vi "Initialise.vi"(8 "error in (no error)":errorcluster, 9 "Current Loop Rate (usec)":u32, 10 "frame":string="/world", 11 "MF3 in":refnum<class "MF3.lvclass">) -> (0 "error out":errorcluster, 3 "MF3 out":refnum<class "MF3.lvclass">)   [LabVIEW 2011, in "MF3.lvclass"]
uses:
  MF3.lvclass
  Controls/Drive Status.ctl
  <vilib>/LabVIEW Targets/FPGA/cRIO/cRIO-9505/controls.llb/_nicrio_cRIO-9505_DriveStatus.ctl
  MF3.lvclass/MF3.ctl
  <vilib>/FPGAPlugInAG/NI 9157/niLvFpga_Open_NI 9157.vi
  <vilib>/Utility/error.llb/Error Cluster From Error Code.vi
  <vilib>/rvi/errors/niLvFpgaAdjustHostInterfaceError.vi
  <vilib>/rvi/interface/nirviOpenFPGA/nirviOpenFPGA.xnode
  FPGA Bitfiles/MotorsInterface.lvbitx
  <vilib>/rvi/interface/nirviReadWriteControl/nirviReadWriteControl.xnode
  Finger/Finger.lvclass
  NiFpgaLv.dll
panel:
  out "Motors Status":T1[](array[typedef])=[{"Status"=enum."Enabled", "Vsup Present"=FALSE, "Drive Fault"=FALSE, "Temp Fault"=FALSE}, {"Status"=enum."Enabled", "Vsup Present"=FALSE, "Drive Fault"=FALSE, "Temp Fault"=FALSE}, {"Status"=enum."Enabled", "Vsup Present"=FALSE, "Drive Fault"=FALSE, "Temp Fault"=FALSE}, {"Status"=enum."Enabled", "Vsup Present"=FALSE, "Drive Fault"=FALSE, "Temp Fault"=FALSE}, {"Status"=enum."Enabled", "Vsup Present"=FALSE, "Drive Fault"=FALSE, "Temp Fault"=FALSE}, {"Status"=enum."Enabled", "Vsup Present"=FALSE, "Drive Fault"=FALSE, "Temp Fault"=FALSE}, {"Status"=enum."Enabled", "Vsup Present"=FALSE, "Drive Fault"=FALSE, "Temp Fault"=FALSE}, {"Status"=enum."Enabled", "Vsup Present"=FALSE, "Drive Fault"=FALSE, "Temp Fault"=FALSE}, {"Status"=enum."Enabled", "Vsup Present"=FALSE, "Drive Fault"=FALSE, "Temp Fault"=FALSE}, {"Status"=enum."Enabled", "Vsup Present"=FALSE, "Drive Fault"=FALSE, "Temp Fault"=FALSE}]
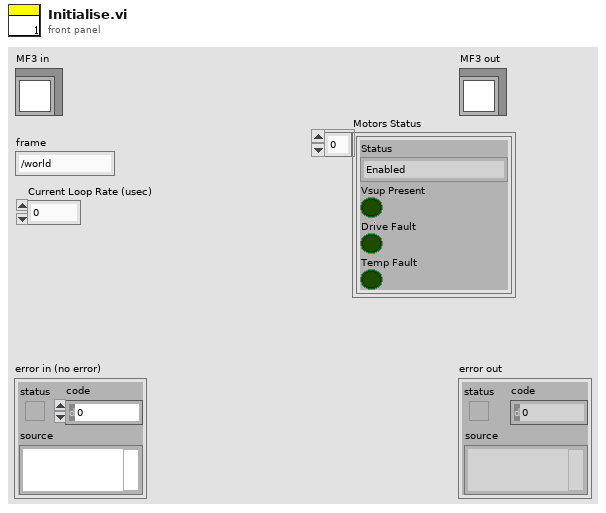
[diagram p1: front panel]
types:
  T1 = typedef "Drive Status.ctl" = cluster{"Status":T2, "Vsup Present":bool, "Drive Fault":bool, "Temp Fault":bool}
  T2 = typedef "_nicrio_cRIO-9505_DriveStatus.ctl" = enum8{"Enabled", "Disabled", "Disabled by Drive Fault", "Disabled by Temp. Fault", "Disabled by E-Stop", "Unknown"}
  T3 = typedef "Dynamic Parameters.ctl" = cluster{"gear_ratios":sgl[]}
  T4 = typedef "NI_Robotics_Link.lvclass/Joint Type.ctl" = enum16{"Revolute", "Prismatic"}
  T5 = typedef "5-bar Side.ctl" = enum16{"Left", "Right"}
  T6 = cluster{"Thumb":cluster{"k":sgl[][], "p":sgl[][], "T0":sgl[][], "types":T4[], "side":T5}, "Middle":cluster{"k":sgl[][], "p":sgl[][], "T0":sgl[][], "types":T4[], "side":T5}, "Index":cluster{"k":sgl[][], "p":sgl[][], "T0":sgl[][], "types":T4[], "side":T5}}
  T7 = cluster{"k":sgl[][], "p":sgl[][], "T0":sgl[][], "types":T4[], "side":T5}
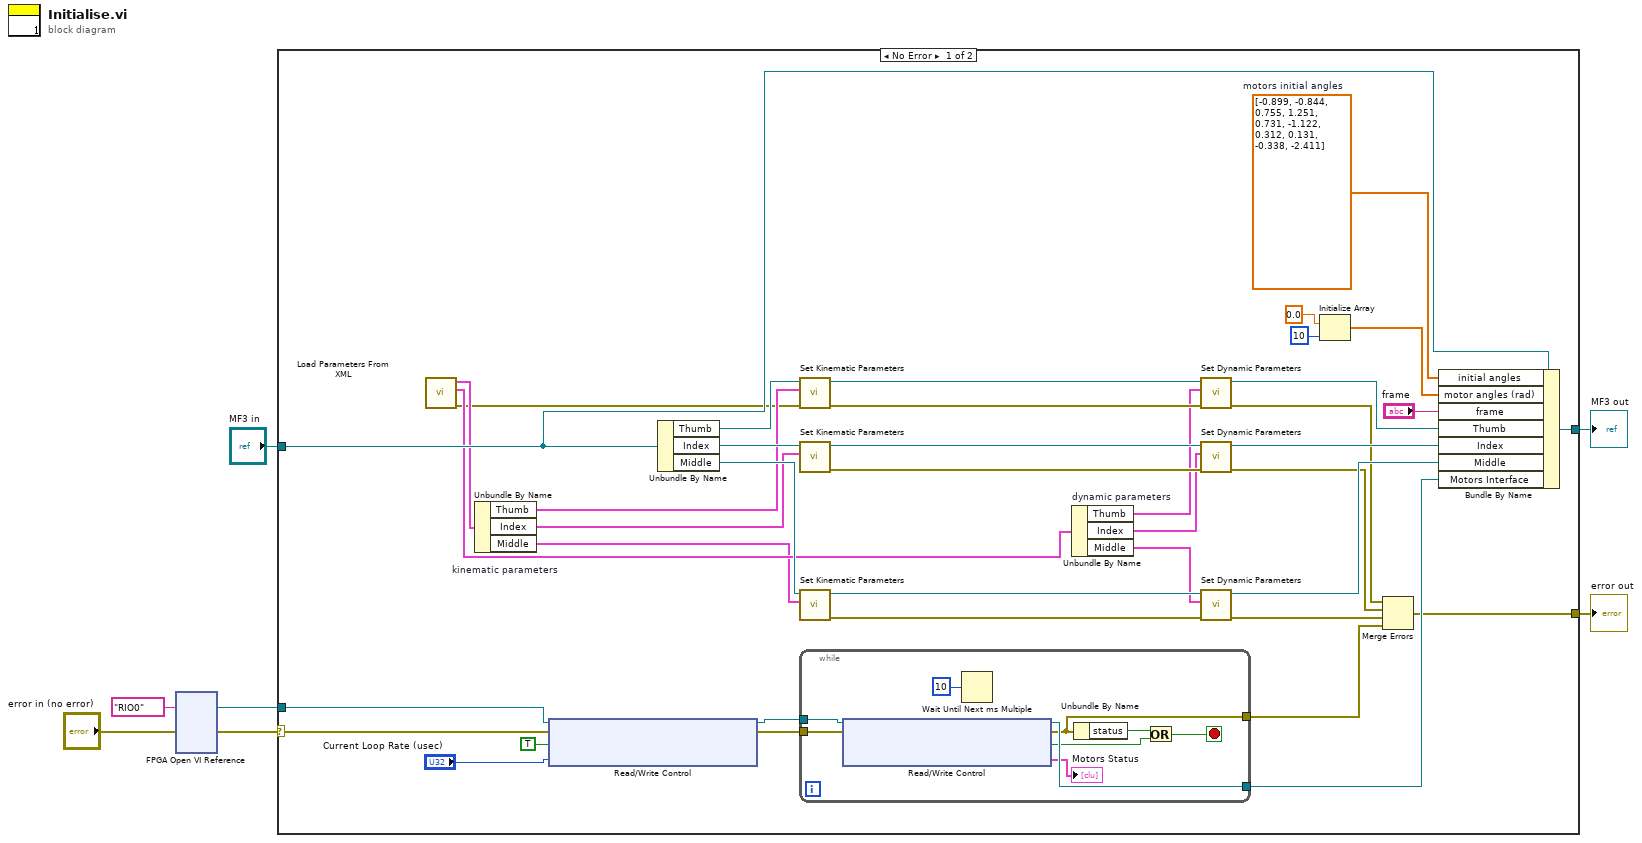
[diagram p0: block diagram]
diagram:
  n1 = xnode "FPGA Open VI Reference"("error in"="error in (no error)", "resource name"=tag "RIO0") -> ("FPGA VI Reference Out"=w2:refnum<k20>, "error out"=w3:errorcluster)
  n2 = case shown="No Error" w3 {
    selector: w3 -> [w41 w58]
    tunnel: [w11 w58] -> w7
    tunnel: [w43 w57] -> w5
    tunnel: "MF3 in" -> [w39 w57]
    tunnel: w2 -> [w47 _]
    frame No Error {
      w23 = dbl[] [-0.899, -0.844, 0.755, 1.251, 0.731, -1.122, 0.312, 0.131, -0.338, -2.411]  # motors initial angles
      n3 = call "Load Parameters From XML.vi"() -> ("error out"=w13:errorcluster, "dynamic parameters"=w21:cluster{"Thumb":T3, "Middle":T3, "Index":T3}, "kinematic parameters"=w17:T6)  [unwired: 9 in]
      n4 = Unbundle By Name "kinematic parameters"(w17) -> ("Thumb"=w16:T7, "Index"=w15:T7, "Middle"=w14:T7)
      n5 = xnode "Read/Write Control"("FPGA VI Reference In"=w47, "error in"=w41, "Enable Motors"=TRUE, "Rate (usec)"="Current Loop Rate (usec)") -> ("FPGA VI Reference Out"=w45:refnum<k20>, "error out"=w44:errorcluster)
      n6 = Unbundle By Name(w39) -> ("Thumb"=w38:refnum<class "Finger.lvclass">, "Index"=w28:refnum<class "Finger.lvclass">, "Middle"=w27:refnum<class "Finger.lvclass">)
      n7 = call "Set Kinematic Parameters.vi"("error in (no error)"=w13, "kinematic parameters"=w16, "Finger in"=w38) -> ("error out"=w36:errorcluster, "Finger out"=w35:refnum<class "Finger.lvclass">)  [unwired: 7 in]
      n8 = call "Set Kinematic Parameters.vi"("kinematic parameters"=w15, "Finger in"=w28) -> ("error out"=w32:errorcluster, "Finger out"=w22:refnum<class "Finger.lvclass">)  [unwired: 8 in]
      n9 = call "Set Kinematic Parameters.vi"("kinematic parameters"=w14, "Finger in"=w27) -> ("error out"=w30:errorcluster, "Finger out"=w31:refnum<class "Finger.lvclass">)  [unwired: 8 in]
      n10 = while {
        tunnel: w45 -> [w56]
        tunnel: w44 -> [w55]
        tunnel: [w54] -> w34
        tunnel: [w51] -> w12
        stop <- w49 stop-if-true
        n11 = xnode "Read/Write Control"("FPGA VI Reference In"=w56, "error in"=w55) -> ("FPGA VI Reference Out"=w54:refnum<k20>, "error out"=w51:errorcluster, "All Enabled"=w52:bool, "Motors Status"=→"Motors Status":T1[])
        n12 = Wait Until Next ms Multiple(millisecond multiple=u32 10) -> ()  [unwired: 1 out]
        n13 = Unbundle By Name(w51) -> ("status"=w50:bool)
        n14 = Or(x=w50, y=w52) -> (x .or. y?=w49:bool)
      }
      n15 = Unbundle By Name "dynamic parameters"(w21) -> ("Thumb"=w20:T3, "Index"=w18:T3, "Middle"=w19:T3)
      n16 = call "Set Dynamic Parameters.vi"("error in (no error)"=w36, "dynamic parameters"=w20, "Finger in"=w35) -> ("error out"=w8:errorcluster, "Finger out"=w37:refnum<class "Finger.lvclass">)  [unwired: 7 in]
      n17 = call "Set Dynamic Parameters.vi"("error in (no error)"=w32, "dynamic parameters"=w18, "Finger in"=w22) -> ("error out"=w9:errorcluster, "Finger out"=w33:refnum<class "Finger.lvclass">)  [unwired: 7 in]
      n18 = call "Set Dynamic Parameters.vi"("error in (no error)"=w30, "dynamic parameters"=w19, "Finger in"=w31) -> ("error out"=w10:errorcluster, "Finger out"=w29:refnum<class "Finger.lvclass">)  [unwired: 7 in]
      n19 = Initialize Array(0.0 ("element"), 10 ("dimension size")) -> (w24:dbl[])
      n20 = Merge Errors(w8, w9, w10, w12) -> (w11:errorcluster)
      n21 = Bundle By Name(cluster=w39, "initial angles"=w23, "motor angles (rad)"=w24, "frame"="frame", "Thumb"=w37, "Index"=w33, "Middle"=w29, "Motors Interface"=w34) -> (w43:refnum<class "MF3.lvclass">)
    }
    frame Error {
    }
  }
  "error out" <- w7
  "MF3 out" <- w5
